vi "save report as PDF 2011.vi"() -> ()   [LabVIEW 2017]
uses:
  <vilib>/Utility/NIReport.llb/NI_report.lvclass
  <vilib>/Utility/NIReport.llb/Excel/NI_Excel.lvclass
  <vilib>/Utility/NIReport.llb/Word/NI_Word.lvclass
panel:
  in  "Report file path":path=path "D:/Customer stuff/1944517 Tom Frei/test.xlsx"
  in  "Report Type":T1(ring)=enum."Excel"
  # "Instructions:\n1) Browse for an existing Word or Excel document\n2) Select the appropriate Report Type\n3) Run the VI. It will save the document as a PDF \n     as \"LabVIEW Save.pdf\" in the same folder as \n     the original report."
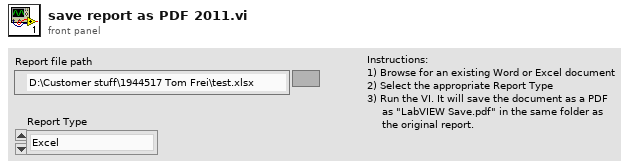
[diagram p1: front panel]
types:
  T1 = enum16{"Standard Report", "HTML", "Word", "Excel"}
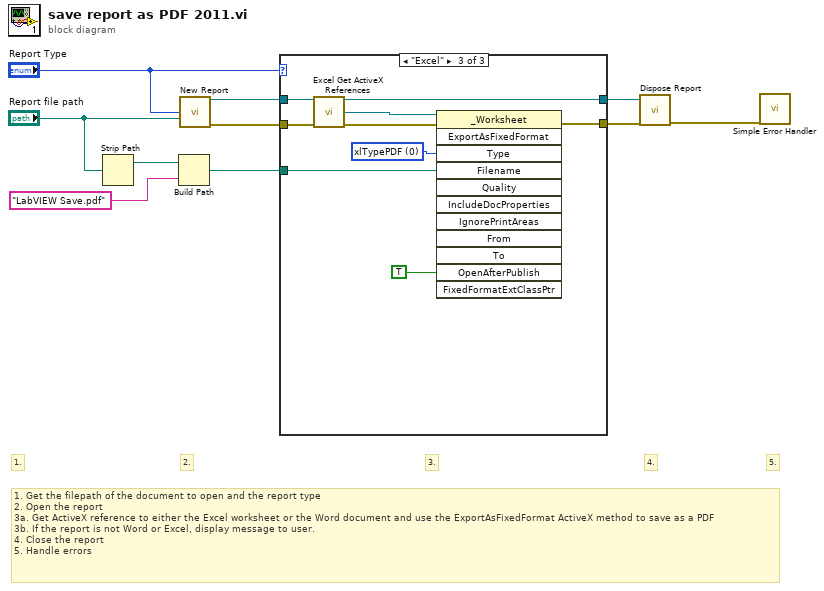
[diagram p0: block diagram]
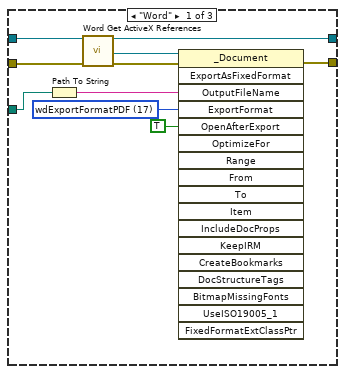
[diagram p2: hidden frame]
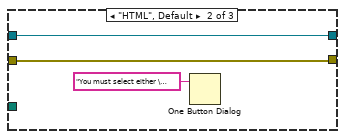
[diagram p3: hidden frame]
diagram:
  # "1. Get the filepath of the document to open and the report type\n2. Open the report\n3a. Get ActiveX reference to either the Excel worksheet or the Word document and use the ExportAsFixedFormat ActiveX method to save as a PDF \n3b. If the report is not Word or Excel, display message to user.\n4. Close the report\n5. Handle errors"
  # "5."
  # "4."
  # "3."
  # "2."
  # "1."
  n1 = Strip Path(path="Report file path") -> (stripped path=w8:path)  [unwired: 1 out]
  n2 = Build Path(base path=w8, name or relative path="LabVIEW Save.pdf") -> (appended path=w6:path)
  n3 = call <vilib>:"New Report.vi"("report type"="Report Type", "template (empty)"="Report file path") -> ("report out"=w10:refnum<class "NI_report.lvclass">, "error out"=w3:errorcluster)  [unwired: 12 in]
  n4 = case shown="\"Excel\"" "Report Type" {
    tunnel: w10 -> [w20 w23 w31]
    tunnel: w6 -> [w17 _ w29]
    tunnel: [w19 w23 w27] -> w5
    tunnel: w3 -> [w14 w21 w26]
    tunnel: [w12 w21 w24] -> w2
    frame "Word" {
      w15 = 17 items=["wdExportFormatPDF"=17, "wdExportFormatXPS"=18] ("ExportFormat")
      n5 = Path To String(path=w17) -> (string=w16:string)
      n6 = call <vilib>:"Word Get ActiveX References.vi"("report in"=w20, "error in (no error)"=w14) -> ("report out"=w19:refnum<class "NI_report.lvclass">, "Word._Document"=w18:refnum<k7>, "error out"=w13:errorcluster)  [unwired: 7 in, 4 out]
      n7 = invoke class="_Document" method="ExportAsFixedFormat"(reference=w18, error in=w13, "OutputFileName"=w16, "ExportFormat"=w15, "OpenAfterExport"=TRUE) -> (error out=w12:errorcluster)  [unwired: 13 in, 17 out]
    }
    frame "HTML", Default {
      n8 = One Button Dialog(message="You must select either \"Word\" or \"Excel\" as the Report Type.") -> ()  [unwired: 1 in, 1 out]
    }
    frame "Excel" {
      w30 = 0 items=["xlTypePDF", "xlTypeXPS"] ("Type")
      n9 = call <vilib>:"Excel Get ActiveX References.vi"("report in"=w31, "error in (no error)"=w26) -> ("report out"=w27:refnum<class "NI_report.lvclass">, "Excel._Worksheet"=w32:refnum<k7>, "error out"=w25:errorcluster)  [unwired: 7 in, 4 out]
      n10 = invoke class="_Worksheet" method="ExportAsFixedFormat"(reference=w32, error in=w25, "Type"=w30, "Filename"=w29, "OpenAfterPublish"=TRUE) -> (error out=w24:errorcluster)  [unwired: 7 in, 11 out]
    }
  }
  n11 = call-dynamic "Dispose Report.vi"("report in"=w5, "error in (no error)"=w2) -> ("error out"=w1:errorcluster)  [unwired: 13 in]
  n12 = call <vilib>:"Simple Error Handler.vi"("error in (no error)"=w1) -> ()  [unwired: 4 in, 5 out]
